vi "Set up chart.vi"(10 "chart reference":refnum<vi>, 11 "Sampling data":T1={"Channels"=[], "Sampling freq"=0, "Output freq"=0, "Update freq"=0, "Steps per rev"=0, "Counts per rev"=0, "Amplifier"="", "Motor driver"="", "Step bit"=0, "Max speed"=0.0, "Max accel"=0.0, "Pos gain"=0.0, "Vel gain"=0.0, "counter"="Dev1/ctr0"} {"Channels"."Hi cutoff" items=["500"=500.0, "1k"=1000.0, "5k"=5000.0, "10k"=10000.0, "20k"=20000.0]; "Channels"."Lo cutoff" items=["0.1"=0.1, "1"=1.0, "10"=10.0, "100"=100.0, "300"=300.0]; "Channels"."Gain" items=["x100"=100, "x1000"=1000, "x10000"=10000]}) -> ()   [LabVIEW 2012]
uses:
  Sampling info.ctl
  Channel.ctl
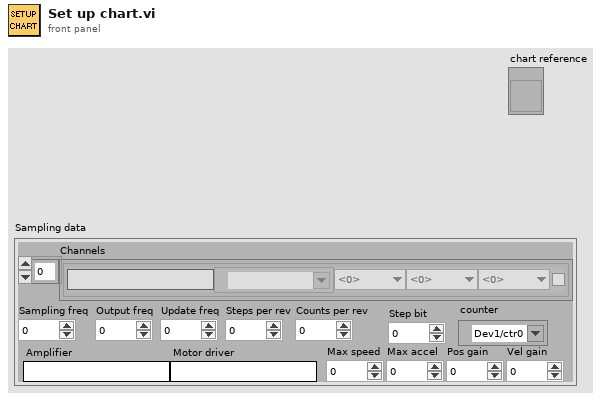
[diagram p1: front panel]
types:
  T1 = typedef "Sampling info.ctl" = cluster{"Channels":T2[], "Sampling freq":i32, "Output freq":i32, "Update freq":i32, "Steps per rev":i32, "Counts per rev":i32, "Amplifier":string, "Motor driver":string, "Step bit":u8, "Max speed":dbl, "Max accel":dbl, "Pos gain":dbl, "Vel gain":dbl, "counter":tag}
  T2 = typedef "Channel.ctl" = cluster{"Name":string, "Chan":tag, "Gain":u16, "Lo cutoff":dbl, "Hi cutoff":dbl, "Notch":bool}
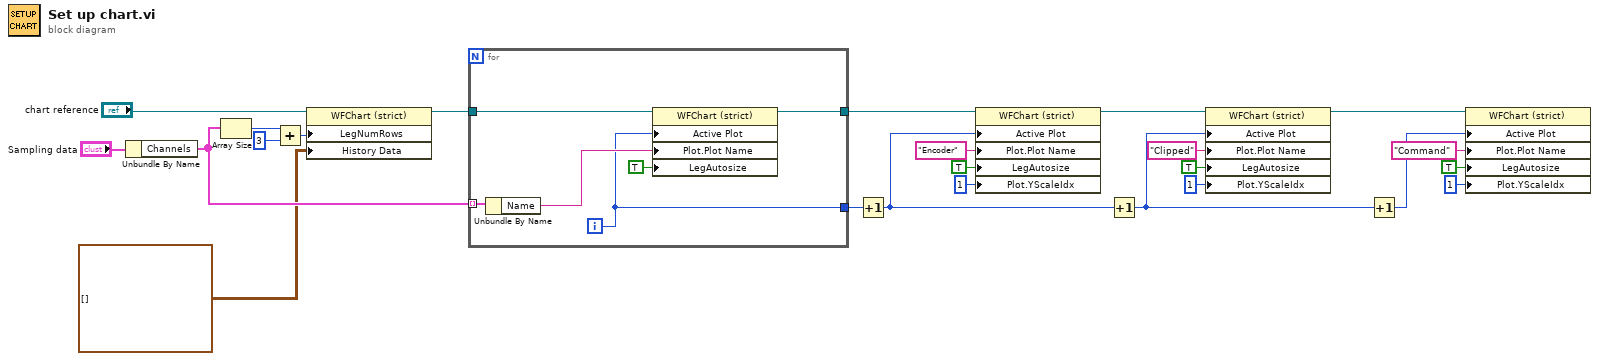
[diagram p0: block diagram]
diagram:
  n1 = Unbundle By Name("Sampling data") -> ("Channels"=w18:T2[])
  n2 = Array Size(array=w18) -> (size(s)=w10:i32)
  n3 = Add(x=w10, y=3) -> (x+y=w16:i32)
  n4 = property class="WFChart (strict)"(reference="chart reference", "LegNumRows"=w16, "History Data"=waveform(dbl)[][] []) -> (reference out=w17:refnum<vi>)  [unwired: 1 in, 1 out]
  n5 = for {
    tunnel: w17 -> [w30]
    tunnel: w18 -> [w29] mode=indexing
    tunnel: [w26] -> w22
    tunnel: [w25] -> w21
    i -> [w25]
    n6 = Unbundle By Name(w29) -> ("Name"=w28:string)
    n7 = property class="WFChart (strict)"(reference=w30, "Active Plot"=w25, "Plot.Plot Name"=w28, "LegAutosize"=TRUE ("Legend:Autosize")) -> (reference out=w26:refnum<vi>)  [unwired: 1 in, 1 out]
  }
  n8 = Increment(x=w21) -> (x+1=w12:i32)
  n9 = property class="WFChart (strict)"(reference=w22, "Active Plot"=w12, "Plot.Plot Name"="Encoder", "LegAutosize"=TRUE ("Legend:Autosize"), "Plot.YScaleIdx"=u32 1 ("Plot.Y Scale Index")) -> (reference out=w11:refnum<vi>)  [unwired: 1 in, 1 out]
  n10 = Increment(x=w12) -> (x+1=w1:i32)
  n11 = property class="WFChart (strict)"(reference=w11, "Active Plot"=w1, "Plot.Plot Name"="Clipped", "LegAutosize"=TRUE ("Legend:Autosize"), "Plot.YScaleIdx"=u32 1 ("Plot.Y Scale Index")) -> (reference out=w2:refnum<vi>)  [unwired: 1 in, 1 out]
  n12 = Increment(x=w1) -> (x+1=w6:i32)
  n13 = property class="WFChart (strict)"(reference=w2, "Active Plot"=w6, "Plot.Plot Name"="Command", "LegAutosize"=TRUE ("Legend:Autosize"), "Plot.YScaleIdx"=u32 1 ("Plot.Y Scale Index")) -> ()  [unwired: 1 in, 2 out]
